vi "DLL_Path.vi"() -> ()   [LabVIEW 2014]
panel:
  in  "DLL_Path":path
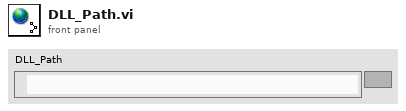
[diagram p1: front panel]
diagram:
